vi "JSON ReadString.vi"(8 "error in (no error)":errorcluster, 9 "Key":string, 11 "JSON":string) -> (0 "error out":errorcluster, 2 "Value":string)   [LabVIEW 2020, in "Error Provider API.lvlib"]
uses:
  <vilib>/NI VeriStand/Error Provider API/Error Provider API.lvlib
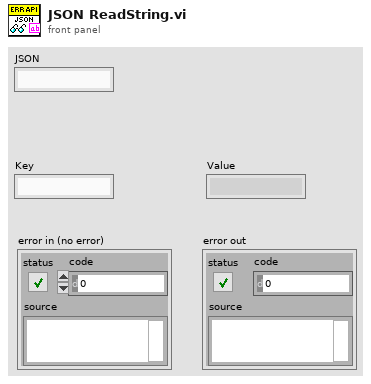
[diagram p1: front panel]
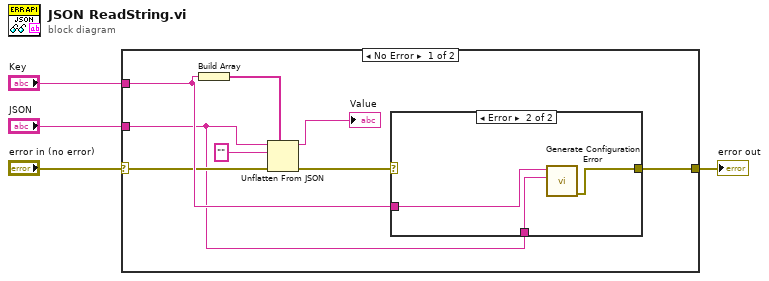
[diagram p0: block diagram]
diagram:
  n1 = case shown="No Error" "error in (no error)" {
    selector: "error in (no error)" -> [w6 w17]
    tunnel: "JSON" -> [w5 _]
    tunnel: [w8 w17] -> w3
    tunnel: "Key" -> [w7 _]
    frame No Error {
      n2 = Build Array(w7) -> (w12:string[])
      n3 = Unflatten From JSON(path=w12, JSON string=w5, type and defaults="", error in (no error)=w6) -> (value=→"Value":string, error out=w9:errorcluster)  [unwired: 3 in]
      n4 = case shown="Error" w9 {
        selector: w9 -> [w13 _]
        tunnel: [w13 w14] -> w8
        tunnel: w7 -> [_ w15]
        tunnel: w5 -> [_ w16]
        frame No Error {
        }
        frame Error {
          n5 = call <vilib>:"Generate Configuration Error.vi"("JSON"=w16, "Key"=w15) -> ("error out"=w14:errorcluster)  [unwired: 9 in]
        }
      }
    }
    frame Error {
    }
  }
  "error out" <- w3
